vi "File Page.vi"(8 "error in (no error)":errorcluster, 11 "Node Ptr":T1 format="%.0x") -> (0 "error out":errorcluster)   [LabVIEW 2027, in "Embedded Data Logger System Explorer.lvlib"]
uses:
  Embedded Data Logger System Explorer.lvlib
  <vilib>/NI VeriStand/Custom Device API/Custom Device Item Ref.ctl
  <vilib>/NI VeriStand/Custom Device API/Custom Device Target Type.ctl
  Shared/Segment Files By.ctl
  <vilib>/NI VeriStand/Custom Device API/Get Item Property (Boolean).vi
  <vilib>/NI VeriStand/Custom Device API/Custom Device API.lvlib
  Scripting/Embedded Data Logger Scripting.lvlib
  Shared/Embedded Data Logger Shared.lvlib
panel:
  in  "Append Waveform Properties":bool caption="Open Log File during Initialization"
  in  "Segment Files By":u16(ring) caption="Based on" items=["Time span (s)", "File size (MB)"]
  in  "Segment File Size":u32=10 caption="Create new file when the time duration exceeds"
  in  "Segment Files":bool caption="Segment into Multiple Files"
  in  "Archive Files":bool caption="Archive Oldest Log Files"
  in  "Archive Directory":path
  in  "Auto Open":bool caption="Open Log File during Initialization"
  in  "Header 4":cluster{"Section Name":string}={"Section Name"="Log File Specification"}
  out "Example Log File Path":path
  in  "Timestamp":bool
  in  "Log File Directory":path
  in  "Pretrigger Samples":i32=100
  in  "Pretrigger":bool
  in  "Header 3":cluster{"Section Name":string}={"Section Name"="Pretrigger Specification"}
  in  "Header":cluster{"Section Name":string}={"Section Name"="Data Log File Settings"}
  in  "Description":string
  in  "Name":string
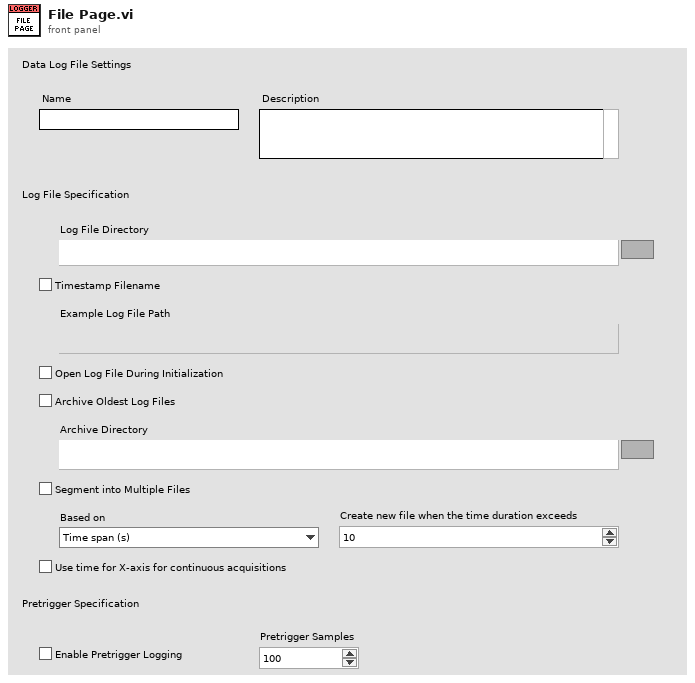
[diagram p1: front panel]
types:
  T1 = typedef "Custom Device API.lvlib/Custom Device Item Ref.ctl" = u64
  T2 = typedef "Custom Device API.lvlib/Custom Device Target Type.ctl" = enum16{"PharLap", "VxWorks", "Windows", "Linux_32_ARM", "Linux_x64"}
  T3 = typedef "Embedded Data Logger Shared.lvlib/Segment Files By.ctl" = enum16{"Time", "Size"}
  T4 = enum8{"Enabled", "Disabled", "Disabled and Grayed Out"}
  T5 = typedef "Custom Device API.lvlib/Custom Device Commands.ctl" = enum16{"Default", "Item renamed", "Shutdown", "Dynamic button pressed"}
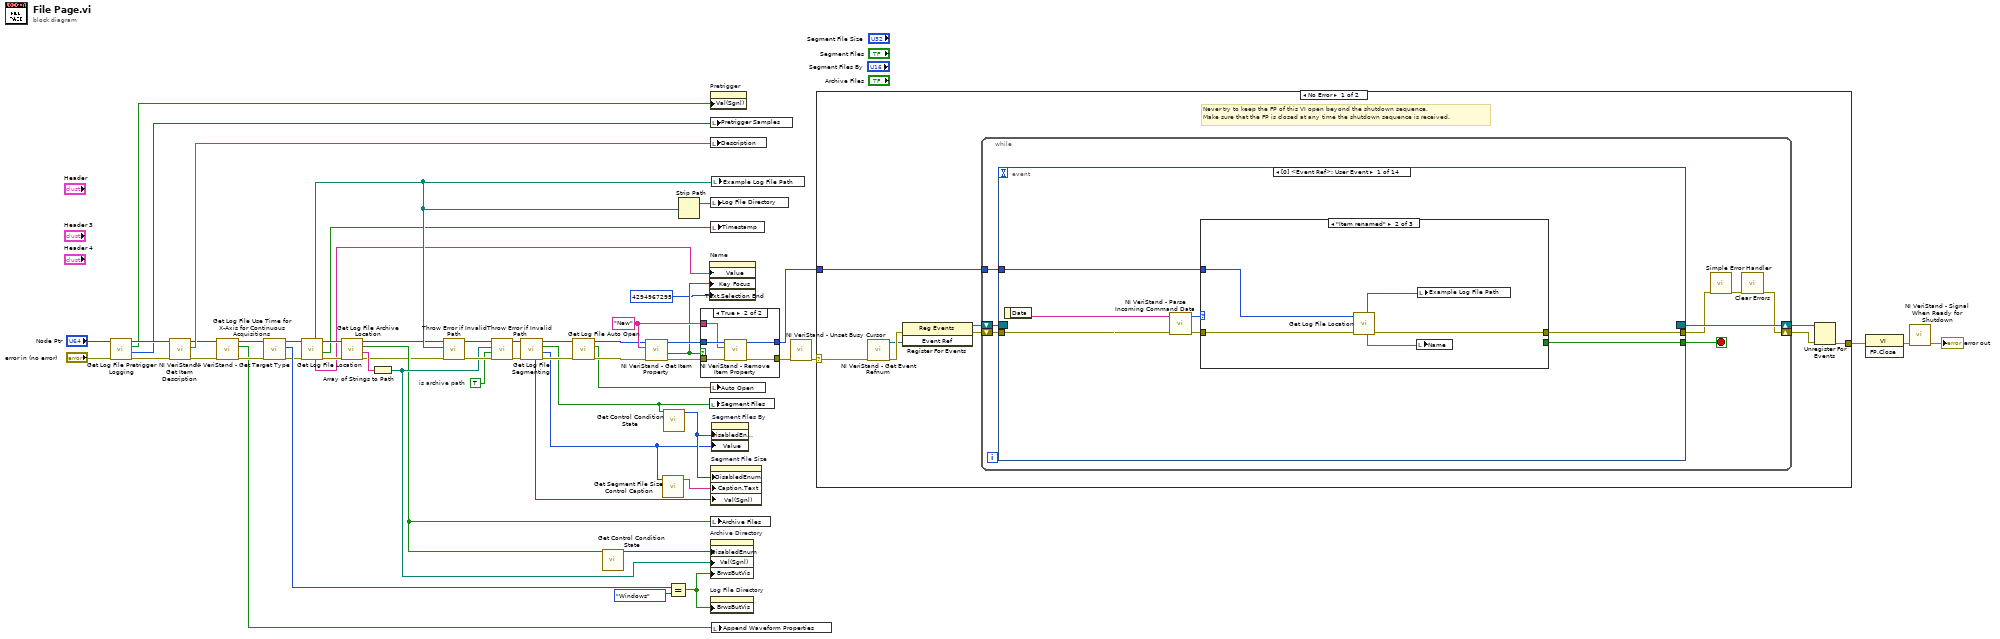
[diagram p0: block diagram]
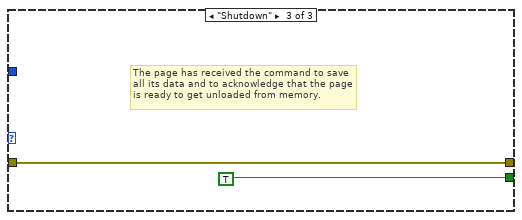
[diagram p4: hidden frame]
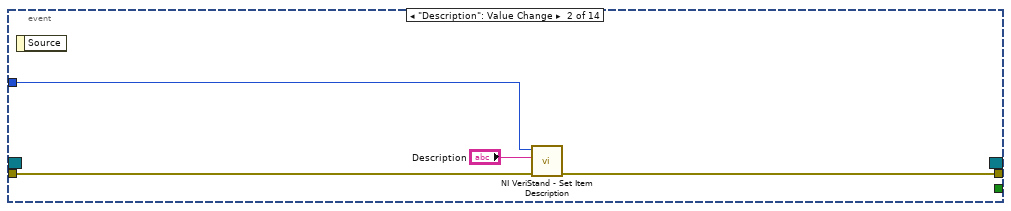
[diagram p5: hidden frame]
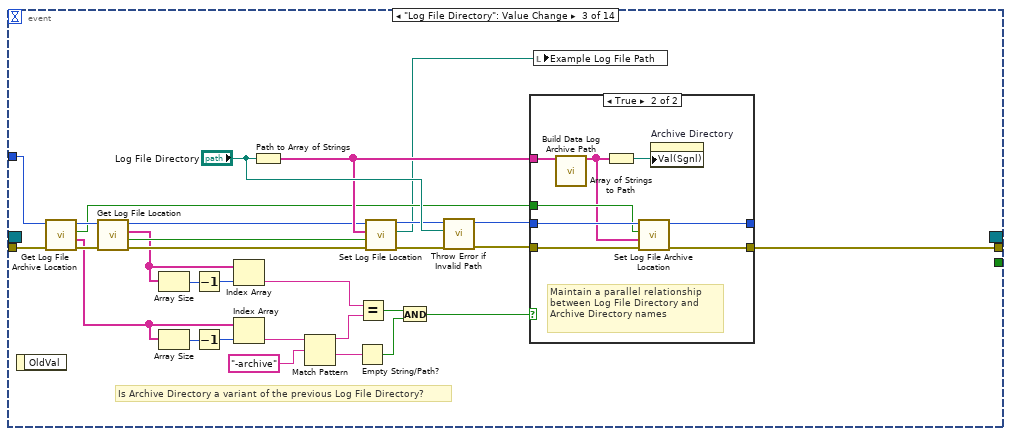
[diagram p6: hidden frame]
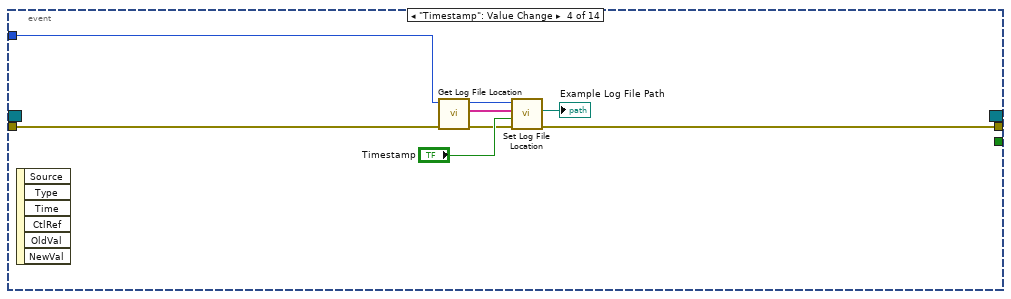
[diagram p8: hidden frame]
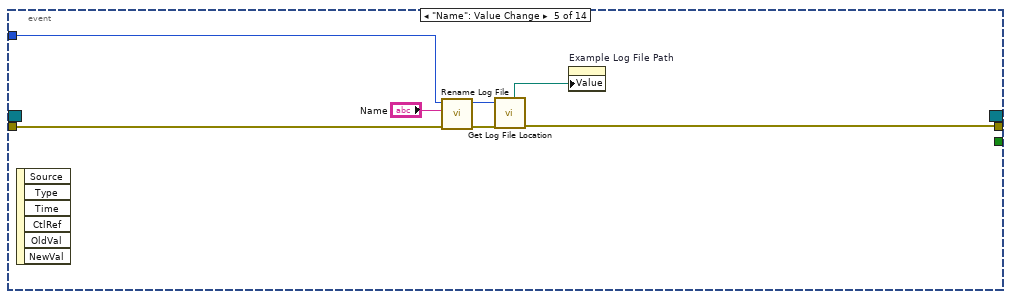
[diagram p9: hidden frame]
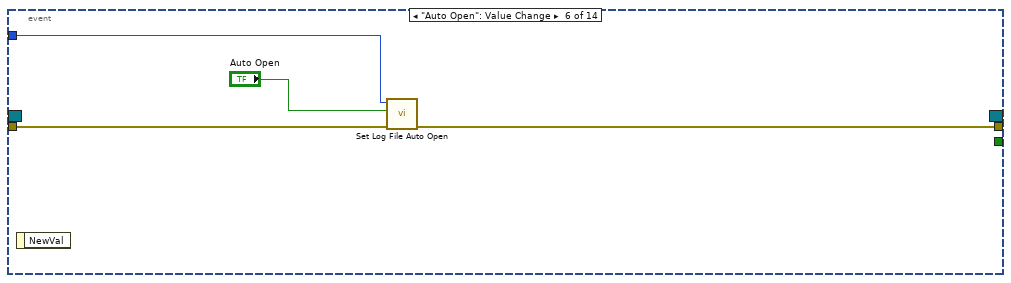
[diagram p10: hidden frame]
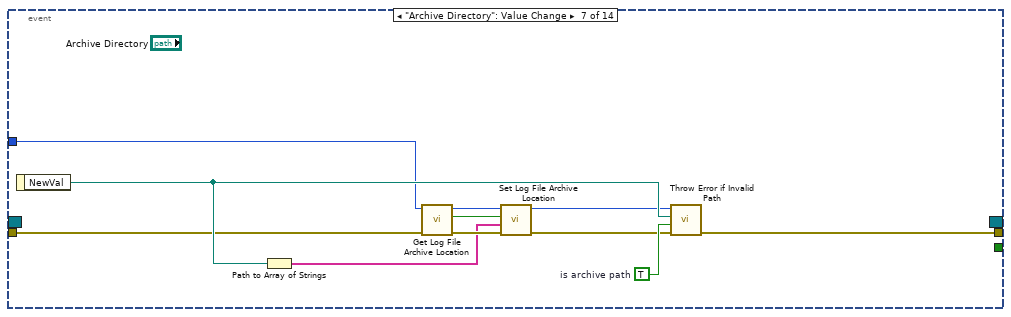
[diagram p11: hidden frame]
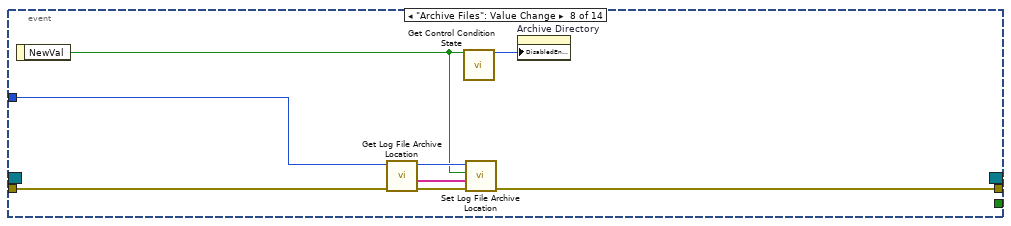
[diagram p12: hidden frame]
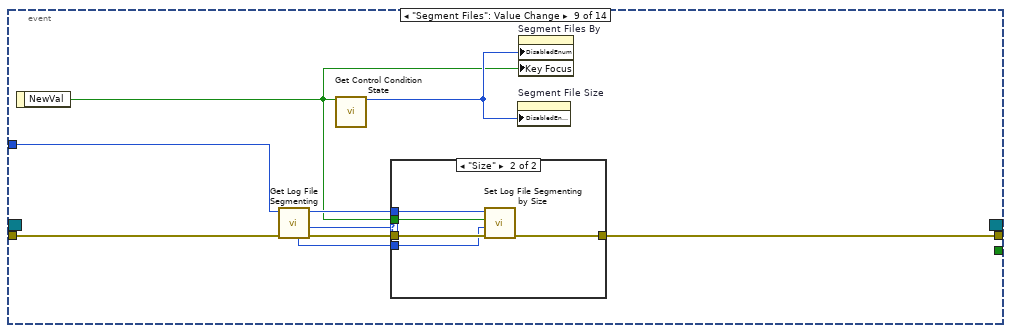
[diagram p13: hidden frame]
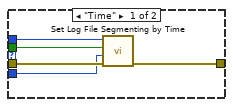
[diagram p14: hidden frame]
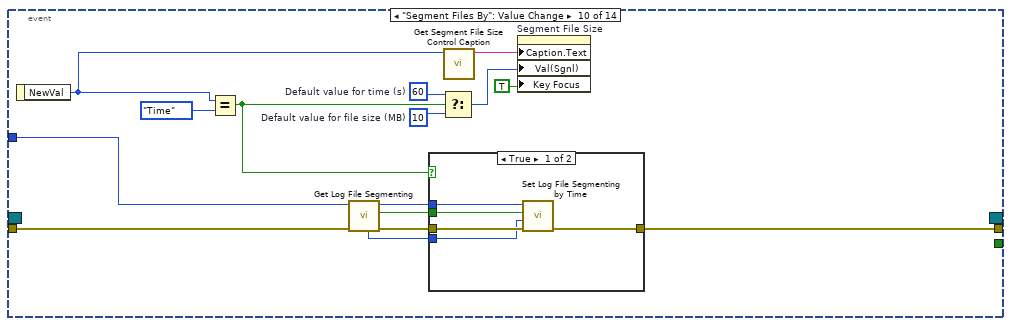
[diagram p15: hidden frame]
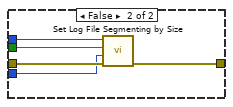
[diagram p16: hidden frame]
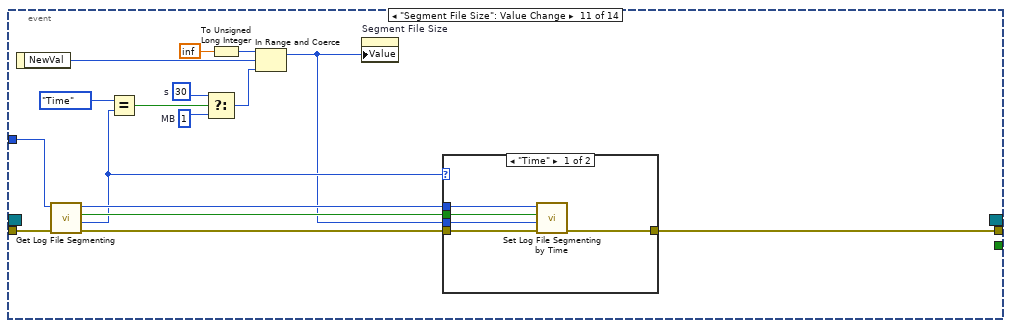
[diagram p17: hidden frame]
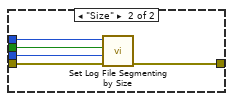
[diagram p18: hidden frame]
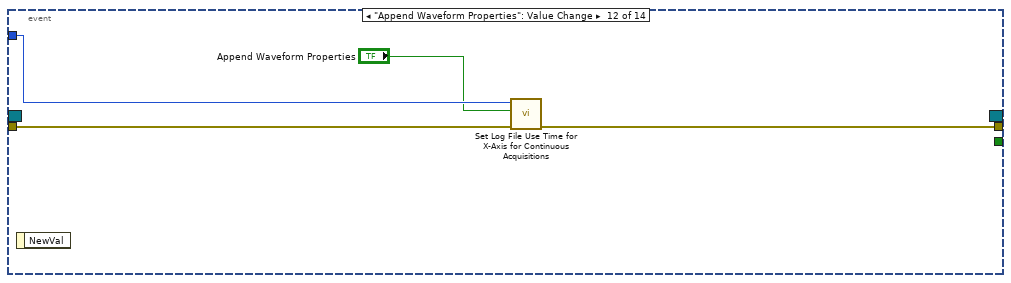
[diagram p19: hidden frame]
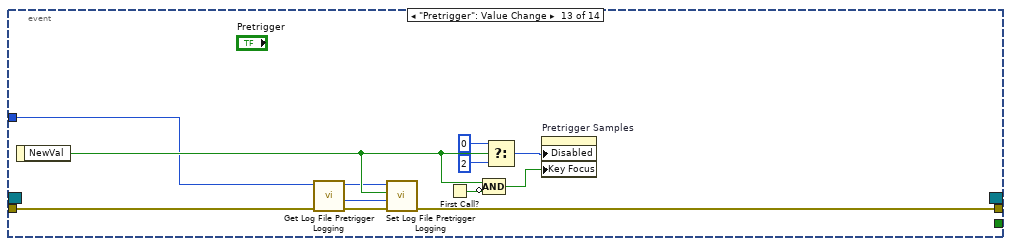
[diagram p20: hidden frame]
diagram:
  w27 = TRUE  # is archive path
  w47 = "New" ("Property Name")
  n1 = call "Get Log File Pretrigger Logging.vi"("error in"="error in (no error)", "log file in"="Node Ptr") -> ("error out"=w3:errorcluster, "pretrigger samples"=w1:i32, "pretrigger logging"=w2:bool, "log file out"=w6:T1)  [unwired: 6 in]
  n2 = call <vilib>:"NI VeriStand - Get Item Description.vi"("error in (no error)"=w3, "Item Ref in"=w6) -> ("error out"=w25:errorcluster, "Description"=w51:string, "Item Ref out"=w26:T1)  [unwired: 7 out]
  n3 = call "Get Log File Use Time for X-Axis for Continuous Acquisitions.vi"("error in"=w25, "log file in"=w26) -> ("error out"=w23:errorcluster, "use time for x-axis for continuous acquisitions"=w22:bool, "log file out"=w24:T1)  [unwired: 7 in]
  n4 = call <vilib>:"NI VeriStand - Get Target Type.vi"("error in (no error)"=w23, "Item Ref in"=w24) -> ("error out"=w17:errorcluster, "Target Type"=w38:T2, "Item Ref out"=w18:T1)  [unwired: 7 in]
  n5 = call "Get Log File Location.vi"("error in (no error)"=w17, "log file in"=w18) -> ("error out"=w15:errorcluster, "timestamp file name"=w9:bool, "log file out"=w16:T1, "base file name"=w11:string, "sample path"=w12:path)  [unwired: 4 in, 1 out]
  n6 = call "Get Log File Archive Location.vi"("error in (no error)"=w15, "log file in"=w16) -> ("error out"=w8:errorcluster, "archive directory parts"=w14:string[], "archive closed log files"=w10:bool, "log file out"=w7:T1)  [unwired: 6 in]
  n7 = Array of Strings to Path(0:w14) -> (2:w13:path)  [unwired: 1 in]
  n8 = call "Throw Error if Invalid Path.vi"("error in"=w8, "file path"=w12, "item reference in"=w7) -> ("error out"=w31:errorcluster, "item reference out"=w30:T1)  [unwired: 7 in]
  n9 = call "Throw Error if Invalid Path.vi"("error in"=w31, "is archive path"=w27, "file path"=w13, "item reference in"=w30) -> ("error out"=w29:errorcluster, "item reference out"=w28:T1)  [unwired: 6 in]
  n10 = call "Get Log File Segmenting.vi"("error in"=w29, "log file in"=w28) -> ("error out"=w35:errorcluster, "file segmenting mode"=w20:T3, "segment into multiple files"=w21:bool, "log file out"=w34:T1, "file length (s) or size (MB)"=w19:u32)  [unwired: 5 in]
  n11 = call "Get Log File Auto Open.vi"("error in"=w35, "log file in"=w34) -> ("error out"=w41:errorcluster, "auto open"=w40:bool, "log file out"=w42:T1)  [unwired: 7 in]
  n12 = call "Get Control Condition State.vi"("Enable"=w10) -> ("Control Condition State"=w39:T4)  [unwired: 14 in]
  n13 = call-poly <vilib>:"NI VeriStand - Get Item Property.vi"("error in (no error)"=w41, "Property Name"=w47, "Item Ref in"=w42) -> ("error out"=w49:errorcluster, "Value"=w44:bool, "Item Ref out"=w48:T1)  [unwired: 5 in, 1 out]
  n14 = call "Get Segment File Size Control Caption.vi"("Segment Files By"=w20) -> ("Segment File Size Caption"=w32:string)  [unwired: 10 in]
  n15 = call "Get Control Condition State.vi"("Enable"=w21) -> ("Control Condition State"=w33:T4)  [unwired: 14 in]
  n16 = Equal?(x=w38, y=Custom_Device_Target_Type."Windows") -> (x = y?=w36:bool)
  n17 = Strip Path(path=w12) -> (stripped path=w50:path)  [unwired: 1 out]
  n18 = case shown="True" w44 {
    tunnel: w49 -> [w57 w61]
    tunnel: [w57 w58] -> w46
    tunnel: w48 -> [w56 w62]
    tunnel: [w56 w59] -> w45
    tunnel: w47 -> [_ w60]
    frame False {
    }
    frame True {
      n19 = call <vilib>:"NI VeriStand - Remove Item Property.vi"("error in (no error)"=w61, "Property Name"=w60, "Item Ref in"=w62) -> ("error out"=w58:errorcluster, "Item Ref out"=w59:T1)  [unwired: 6 in, 1 out]
    }
  }
  n20 = property on="Name" class="Str"("Value"=w11, "Key Focus"=w44, "Text.Selection End"=u32 4294967295 ("Text.Selection:End")) -> ()  [unwired: 2 in, 2 out]
  n21 = local write "Segment Files"(w21) -> ()
  n22 = property on="Pretrigger" class="Bool (strict)"("Val(Sgnl)"=w2) -> ()  [unwired: 2 in, 2 out]
  n23 = local write "Pretrigger Samples"(w1) -> ()
  n24 = local write "Description"(w51) -> ()
  n25 = local write "Auto Open"(w40) -> ()
  n26 = property on="Archive Directory" class="Path"("DisabledEnum"=w39, "Val(Sgnl)"=w13, "BrwsButVis"=w36) -> ()  [unwired: 2 in, 2 out]
  n27 = property on="Log File Directory" class="Path"("BrwsButVis"=w36) -> ()  [unwired: 2 in, 2 out]
  n28 = local write "Log File Directory"(w50) -> ()
  n29 = local write "Timestamp"(w9) -> ()
  n30 = property on="Segment File Size" class="DigNum (strict)"("DisabledEnum"=w33, "Caption.Text"=w32, "Val(Sgnl)"=w19) -> ()  [unwired: 2 in, 2 out]
  n31 = local write "Archive Files"(w10) -> ()
  n32 = local write "Example Log File Path"(w12) -> ()
  n33 = property on="Segment Files By" class="Ring (strict)"("DisabledEnum"=w33, "Value"=w20) -> ()  [unwired: 2 in, 2 out]
  n34 = local write "Append Waveform Properties"(w22) -> ()
  n35 = call <vilib>:"NI VeriStand - Unset Busy Cursor.vi"("error in (no error)"=w46) -> ("error out"=w52:errorcluster)  [unwired: 10 out]
  n36 = case shown="No Error" w52 {
    selector: w52 -> [w63 w277]
    tunnel: [w68 w275] -> w55
    tunnel: w45 -> [w64 _]
    frame No Error {
      # "Never try to keep the FP of this VI open beyond the shutdown sequence.\nMake sure that the FP is closed at any time the shutdown sequence is received."
      n37 = call <vilib>:"NI VeriStand - Get Event Refnum.vi"("error in (no error)"=w63) -> ("error out"=w71:errorcluster, "Event Ref"=w67:refnum<user-event>)  [unwired: 9 out]
      n38 = register-events(error in=w71, w67) -> (reference out=w65:refnum<event-registration>, error out=w66:errorcluster)  [unwired: 1 in]
      n39 = while {
        tunnel: w64 -> [w75]
        shift-right: [w72] -> w69
        shift-left: w66 -> [w78]
        shift-right: [w79] -> w70
        shift-left: w65 -> [w77]
        stop <- w76 stop-if-true
        n40 = event shown="[0] <Event Ref>: User Event" {
          selector: w77 -> [_ _ _ _ _ _ _ _ _ _ _ _ _ _]
          dyn-events: [_ _ _ _ _ _ _ _ _ _ _ _ _ _] -> w79
          timeout: _ -> [_ _ _ _ _ _ _ _ _ _ _ _ _ _]
          tunnel: w78 -> [w86 w97 w107 w144 w153 w156 w163 w172 w180 w204 w225 w249 w262 w267]
          tunnel: [w82 _ _ _ _ _ _ _ _ _ _ _ _ _] -> w76
          tunnel: [w81 w96 w100 w140 w148 w155 w168 w171 w179 w201 w227 w248 w257 w266] -> w74
          tunnel: w75 -> [w80 w98 w108 w141 w147 w157 w162 w170 w181 w203 w226 w250 w253 w265]
          event User Event {
            n41 = event-data() -> ("Data"=w85:string)  [unwired: 1 out]
            n42 = call <vilib>:"NI VeriStand - Parse Incoming Command Data.vi"("error in (no error)"=w86, "Incoming data"=w85) -> ("error out"=w84:errorcluster, "Action"=w83:T5)  [unwired: 8 out]
            n43 = case shown="\"Item renamed\"" w83 {
              tunnel: w84 -> [w87 w90 w93]
              tunnel: [_ _ TRUE] -> w82
              tunnel: [w87 w92 w93] -> w81
              tunnel: w80 -> [_ w91 _]
              frame "Default", Default {
              }
              frame "Item renamed" {
                n44 = call "Get Log File Location.vi"("error in (no error)"=w90, "log file in"=w91) -> ("error out"=w92:errorcluster, "base file name"=w89:string, "sample path"=w88:path)  [unwired: 4 in, 3 out]
                n45 = local write "Name"(w89) -> ()
                n46 = local write "Example Log File Path"(w88) -> ()
              }
              frame "Shutdown" {
                # "The page has received the command to save all its data and to acknowledge that the page is ready to get unloaded from memory."
              }
            }
          }
          event "Description": Value Change {
            n47 = event-data() -> ()  [unwired: 2 out]
            n48 = call <vilib>:"NI VeriStand - Set Item Description.vi"("error in (no error)"=w97, "Description"="Description", "Item Ref in"=w98) -> ("error out"=w96:errorcluster)  [unwired: 8 out]
          }
          event "Log File Directory": Value Change {
            # "Is Archive Directory a variant of the previous Log File Directory?"
            n49 = event-data() -> ()  [unwired: 2 out]
            n50 = call "Get Log File Archive Location.vi"("error in (no error)"=w107, "log file in"=w108) -> ("error out"=w106:errorcluster, "archive directory parts"=w101:string[], "archive closed log files"=w105:bool, "log file out"=w109:T1)  [unwired: 6 in]
            n51 = call "Get Log File Location.vi"("error in (no error)"=w106, "log file in"=w109) -> ("error out"=w117:errorcluster, "timestamp file name"=w118:bool, "directory parts"=w113:string[], "log file out"=w116:T1)  [unwired: 4 in, 2 out]
            n52 = Array Size(array=w113) -> (size(s)=w114:i32)
            n53 = Array Size(array=w101) -> (size(s)=w104:i32)
            n54 = Decrement(x=w114) -> (x-1=w115:i32)
            n55 = Decrement(x=w104) -> (x-1=w103:i32)
            n56 = Index Array(array=w113, index=w115) -> (element=w112:string)
            n57 = Index Array(array=w101, index=w103) -> (element=w102:string)
            n58 = Path to Array of Strings(0:"Log File Directory") -> (2:w119:string[])  [unwired: 1 out]
            n59 = Match Pattern(string=w102, regular expression="-archive") -> (before substring=w127:string, after substring=w124:string)  [unwired: 1 in, 2 out]
            n60 = Empty String/Path?(string/path=w124) -> (empty?=w125:bool)
            n61 = Equal?(x=w112, y=w127) -> (x = y?=w126:bool)
            n62 = call "Set Log File Location.vi"("error in"=w117, "timestamp file name"=w118, "directory parts"=w119, "log file in"=w116) -> ("error out"=w111:errorcluster, "sample path"=w99:path, "log file out"=w110:T1)  [unwired: 5 in]
            n63 = And(x=w126, y=w125) -> (x .and. y?=w123:bool)
            n64 = call "Throw Error if Invalid Path.vi"("error in"=w111, "file path"="Log File Directory", "item reference in"=w110) -> ("error out"=w122:errorcluster, "item reference out"=w121:T1)  [unwired: 7 in]
            n65 = case shown="True" w123 {
              tunnel: w121 -> [w130 w137]
              tunnel: w122 -> [w129 w134]
              tunnel: [w130 w136] -> _
              tunnel: [w129 w135] -> w100
              tunnel: w119 -> [_ w138]
              tunnel: w105 -> [_ w133]
              frame False {
                # "User has deviated from similar naming between log & archive directories. So leave Archive Directory alone."
              }
              frame True {
                # "Maintain a parallel relationship between Log File Directory and Archive Directory names"
                n66 = call "Build Data Log Archive Path.vi"("Log Directory String Array"=w138) -> ("Log Archive Directory String Array"=w132:string[])  [unwired: 14 in]
                n67 = Array of Strings to Path(0:w132) -> (2:w131:path)  [unwired: 1 in]
                n68 = call "Set Log File Archive Location.vi"("error in (no error)"=w134, "archive directory parts"=w132, "archive closed log files"=w133, "log file in"=w137) -> ("error out"=w135:errorcluster, "log file out"=w136:T1)  [unwired: 6 in]
                n69 = property on="Archive Directory" class="Path"("Val(Sgnl)"=w131) -> ()  [unwired: 2 in, 2 out]
              }
            }
            n70 = local write "Example Log File Path"(w99) -> ()
          }
          event "Timestamp": Value Change {
            n71 = event-data() -> ()  [unwired: 7 out]
            n72 = call "Get Log File Location.vi"("error in (no error)"=w144, "log file in"=w141) -> ("error out"=w143:errorcluster, "directory parts"=w146:string[], "log file out"=w142:T1)  [unwired: 4 in, 3 out]
            n73 = call "Set Log File Location.vi"("error in"=w143, "timestamp file name"="Timestamp", "directory parts"=w146, "log file in"=w142) -> ("error out"=w140:errorcluster, "sample path"=→"Example Log File Path":path)  [unwired: 5 in, 1 out]
          }
          event "Name": Value Change {
            n74 = event-data() -> ()  [unwired: 7 out]
            n75 = call "Rename Log File.vi"("error in"=w153, "file name"="Name", "log file in"=w147) -> ("error out"=w152:errorcluster, "log file out"=w151:T1)  [unwired: 7 in]
            n76 = call "Get Log File Location.vi"("error in (no error)"=w152, "log file in"=w151) -> ("error out"=w148:errorcluster, "sample path"=w150:path)  [unwired: 4 in, 4 out]
            n77 = property on="Example Log File Path" class="Path"("Value"=w150) -> ()  [unwired: 2 in, 2 out]
          }
          event "Auto Open": Value Change {
            n78 = event-data() -> ()  [unwired: 2 out]
            n79 = call "Set Log File Auto Open.vi"("error in"=w156, "auto open"="Auto Open", "log file in"=w157) -> ("error out"=w155:errorcluster)  [unwired: 7 in, 1 out]
          }
          event "Archive Directory": Value Change {
            w167 = TRUE  # is archive path
            n80 = event-data() -> ("NewVal"=w166:path)  [unwired: 1 out]
            n81 = Path to Array of Strings(0:w166) -> (2:w161:string[])  [unwired: 1 out]
            n82 = call "Get Log File Archive Location.vi"("error in (no error)"=w163, "log file in"=w162) -> ("error out"=w164:errorcluster, "archive closed log files"=w160:bool, "log file out"=w165:T1)  [unwired: 6 in, 1 out]
            n83 = call "Set Log File Archive Location.vi"("error in (no error)"=w164, "archive directory parts"=w161, "archive closed log files"=w160, "log file in"=w165) -> ("error out"=w159:errorcluster, "log file out"=w158:T1)  [unwired: 6 in]
            n84 = call "Throw Error if Invalid Path.vi"("error in"=w159, "is archive path"=w167, "file path"=w166, "item reference in"=w158) -> ("error out"=w168:errorcluster)  [unwired: 6 in, 1 out]
          }
          event "Archive Files": Value Change {
            n85 = event-data() -> ("NewVal"=w169:bool)  [unwired: 1 out]
            n86 = call "Get Log File Archive Location.vi"("error in (no error)"=w172, "log file in"=w170) -> ("error out"=w174:errorcluster, "archive directory parts"=w173:string[], "log file out"=w175:T1)  [unwired: 6 in, 1 out]
            n87 = call "Get Control Condition State.vi"("Enable"=w169) -> ("Control Condition State"=w176:T4)  [unwired: 14 in]
            n88 = call "Set Log File Archive Location.vi"("error in (no error)"=w174, "archive directory parts"=w173, "archive closed log files"=w169, "log file in"=w175) -> ("error out"=w171:errorcluster)  [unwired: 6 in, 1 out]
            n89 = property on="Archive Directory" class="Path"("DisabledEnum"=w176) -> ()  [unwired: 2 in, 2 out]
          }
          event "Segment Files": Value Change {
            n90 = event-data() -> ("NewVal"=w177:bool)  [unwired: 1 out]
            n91 = call "Get Log File Segmenting.vi"("error in"=w180, "log file in"=w181) -> ("error out"=w184:errorcluster, "file segmenting mode"=w178:T3, "log file out"=w183:T1, "file length (s) or size (MB)"=w182:u32)  [unwired: 5 in, 1 out]
            n92 = call "Get Control Condition State.vi"("Enable"=w177) -> ("Control Condition State"=w185:T4)  [unwired: 14 in]
            n93 = case shown="\"Size\"" w178 {
              tunnel: w184 -> [w190 w194]
              tunnel: [w189 w193] -> w179
              tunnel: w183 -> [w188 w195]
              tunnel: w177 -> [w187 w192]
              tunnel: w182 -> [w186 w191]
              frame "Time" {
                n94 = call "Set Log File Segmenting by Time.vi"("error in"=w190, "file length (s)"=w186, "segment into multiple files"=w187, "log file in"=w188) -> ("error out"=w189:errorcluster)  [unwired: 6 in, 1 out]
              }
              frame "Size" {
                n95 = call "Set Log File Segmenting by Size.vi"("error in"=w194, "file size (MB)"=w191, "segment into multiple files"=w192, "log file in"=w195) -> ("error out"=w193:errorcluster)  [unwired: 6 in, 1 out]
              }
            }
            n96 = property on="Segment File Size" class="DigNum (strict)"("DisabledEnum"=w185) -> ()  [unwired: 2 in, 2 out]
            n97 = property on="Segment Files By" class="Ring (strict)"("DisabledEnum"=w185, "Key Focus"=w177) -> ()  [unwired: 2 in, 2 out]
          }
          event "Segment Files By": Value Change {
            w207 = u32 10  # Default value for file size (MB)
            w209 = u32 60  # Default value for time (s)
            n98 = event-data() -> ("NewVal"=w205:u16)  [unwired: 1 out]
            n99 = Equal?(x=w205, y=Segment_Files_By."Time" ("file segmenting mode")) -> (x = y?=w196:bool)
            n100 = call "Get Log File Segmenting.vi"("error in"=w204, "log file in"=w203) -> ("error out"=w202:errorcluster, "segment into multiple files"=w199:bool, "log file out"=w200:T1, "file length (s) or size (MB)"=w198:u32)  [unwired: 5 in, 1 out]
            n101 = case shown="True" w196 {
              tunnel: w202 -> [w215 w219]
              tunnel: [w214 w218] -> w201
              tunnel: w200 -> [w213 w220]
              tunnel: w199 -> [w212 w217]
              tunnel: w198 -> [w211 w216]
              frame True {
                n102 = call "Set Log File Segmenting by Time.vi"("error in"=w215, "file length (s)"=w211, "segment into multiple files"=w212, "log file in"=w213) -> ("error out"=w214:errorcluster)  [unwired: 6 in, 1 out]
              }
              frame False {
                n103 = call "Set Log File Segmenting by Size.vi"("error in"=w219, "file size (MB)"=w216, "segment into multiple files"=w217, "log file in"=w220) -> ("error out"=w218:errorcluster)  [unwired: 6 in, 1 out]
              }
            }
            n104 = Select(t=w209, s=w196, f=w207) -> (s? t:f=w208:u32)
            n105 = call "Get Segment File Size Control Caption.vi"("Segment Files By"=w205) -> ("Segment File Size Caption"=w210:string)  [unwired: 10 in]
            n106 = property on="Segment File Size" class="DigNum (strict)"("Caption.Text"=w210, "Val(Sgnl)"=w208, "Key Focus"=TRUE) -> ()  [unwired: 2 in, 2 out]
          }
          event "Segment File Size": Value Change {
            w232 = u32 1  # MB
            w233 = u32 30  # s
            n107 = event-data() -> ("NewVal"=w236:u32)  [unwired: 1 out]
            n108 = call "Get Log File Segmenting.vi"("error in"=w225, "log file in"=w226) -> ("error out"=w230:errorcluster, "file segmenting mode"=w223:T3, "segment into multiple files"=w228:bool, "log file out"=w229:T1)  [unwired: 5 in, 1 out]
            n109 = Equal?(x=Segment_Files_By."Time" ("file segmenting mode"), y=w223) -> (x = y?=w222:bool)
            n110 = Select(t=w233, s=w222, f=w232) -> (s? t:f=w231:u32)
            n111 = To Unsigned Long Integer(number=inf) -> (unsigned 32bit integer=w234:u32)
            n112 = In Range and Coerce(upper limit=w234, x=w236, lower limit=w231) -> (coerced(x)=w221:u32)  [unwired: 1 out]
            n113 = property on="Segment File Size" class="DigNum (strict)"("Value"=w221) -> ()  [unwired: 2 in, 2 out]
            n114 = case shown="\"Time\"" w223 {
              tunnel: w230 -> [w241 w245]
              tunnel: [w240 w244] -> w227
              tunnel: w229 -> [w239 w246]
              tunnel: w228 -> [w238 w243]
              tunnel: w221 -> [w237 w242]
              frame "Time" {
                n115 = call "Set Log File Segmenting by Time.vi"("error in"=w241, "file length (s)"=w237, "segment into multiple files"=w238, "log file in"=w239) -> ("error out"=w240:errorcluster)  [unwired: 6 in, 1 out]
              }
              frame "Size" {
                n116 = call "Set Log File Segmenting by Size.vi"("error in"=w245, "file size (MB)"=w242, "segment into multiple files"=w243, "log file in"=w246) -> ("error out"=w244:errorcluster)  [unwired: 6 in, 1 out]
              }
            }
          }
          event "Append Waveform Properties": Value Change {
            n117 = event-data() -> ()  [unwired: 2 out]
            n118 = call "Set Log File Use Time for X-Axis for Continuous Acquisitions.vi"("error in"=w249, "use time for x-axis for continuous acquisitions"="Append Waveform Properties", "log file in"=w250) -> ("error out"=w248:errorcluster)  [unwired: 7 in, 1 out]
          }
          event "Pretrigger": Value Change {
            n119 = event-data() -> ("NewVal"=w258:bool)  [unwired: 1 out]
            n120 = call "Get Log File Pretrigger Logging.vi"("error in"=w262, "log file in"=w253) -> ("error out"=w254:errorcluster, "pretrigger samples"=w251:i32, "log file out"=w252:T1)  [unwired: 6 in, 1 out]
            n121 = call "Set Log File Pretrigger Logging.vi"("error in"=w254, "pretrigger samples"=w251, "pretrigger logging"=w258, "log file in"=w252) -> ("error out"=w257:errorcluster)  [unwired: 6 in, 1 out]
            n122 = First Call?() -> (First Call?: T/F=w255:bool)
            n123 = Compound Arithmetic op=AND(w258, invert w255) -> (w256:bool)
            n124 = Select(t=u8 0, s=w258, f=u8 2 ("t")) -> (s? t:f=w259:u8)
            n125 = property on="Pretrigger Samples" class="DigNum (strict)"("Disabled"=w259, "Key Focus"=w256) -> ()  [unwired: 2 in, 2 out]
          }
          event "Pretrigger Samples": Value Change {
            # "Artificial limit of 10M pretrigger samples."
            n126 = event-data() -> ()  [unwired: 2 out]
            n127 = In Range and Coerce(upper limit=10000000, x="Pretrigger Samples", lower limit=1) -> (coerced(x)=w263:i32, In Range?=w270:bool)
            n128 = call "Get Log File Pretrigger Logging.vi"("error in"=w267, "log file in"=w265) -> ("error out"=w269:errorcluster, "pretrigger logging"=w264:bool, "log file out"=w268:T1)  [unwired: 6 in, 1 out]
            n129 = case shown="False" w270 {
              tunnel: w263 -> [w274 _]
              frame False {
                n130 = local write "Pretrigger Samples"(w274) -> ()
              }
              frame True {
              }
            }
            n131 = call "Set Log File Pretrigger Logging.vi"("error in"=w269, "pretrigger samples"=w263, "pretrigger logging"=w264, "log file in"=w268) -> ("error out"=w266:errorcluster)  [unwired: 6 in, 1 out]
          }
        }
        n132 = call <vilib>:"Simple Error Handler.vi"("error in (no error)"=w74) -> ("error out"=w73:errorcluster)  [unwired: 1 in, 7 out]
        n133 = call <vilib>:"Clear Errors.vi"("error in (no error)"=w73) -> ("error out"=w72:errorcluster)  [unwired: 1 in, 5 out]
      }
      n134 = Unregister For Events(event registration refnum=w70, error in=w69) -> (error out=w68:errorcluster)
    }
    frame Error {
      n135 = call <vilib>:"Simple Error Handler.vi"("error in (no error)"=w277) -> ("error out"=w276:errorcluster)  [unwired: 1 in, 7 out]
      n136 = call <vilib>:"Clear Errors.vi"("error in (no error)"=w276) -> ("error out"=w275:errorcluster)  [unwired: 1 in, 5 out]
    }
  }
  n137 = invoke class="VI" method="FP.Close"(error in=w55) -> (error out=w54:errorcluster)  [unwired: 2 in, 2 out]
  n138 = call <vilib>:"NI VeriStand - Signal When Ready for Shutdown.vi"("error in (no error)"=w54) -> ("error out"=→"error out":errorcluster)  [unwired: 10 out]
